vi "top地址搜索.vi"() -> ()   [LabVIEW 2020]
uses:
  e70b21cd-6488-4bde-bb2b-1088b515f470.vi
  <vilib>/Utility/file.llb/Read Delimited Spreadsheet (string).vi
  <vilib>/Comparison/Equal/Equal Functor/Equal Functor.lvclass
panel:
  in  "file path (dialog if empty) 2":path=path "D:/NI 资源包/2-币猎人-事件状态机930/source/规则大数.txt" caption="文件路径 （空时为对话框）"
  out "子数组 3":string[](array[string])
  out "子数组 2":string[](array[string])
  out "数值 2":i32
  out "添加的路径":path
  in  "停止":bool
  out "地址":string
  out "数组":string[][](array[string])
  out "数值":i32
  out "文件名":string[](array[string])
  out "路径输出":path
  in  "路径":path=path "D:/NI 资源包/2-币猎人-事件状态机930/source/网址私钥获取/btc搜寻器/top 账号数据"
  out "index of element":i32 caption="元素索引"
  out "子数组":string[](array[string])
  out "all rows":string[][](array[string]) caption="所有行"
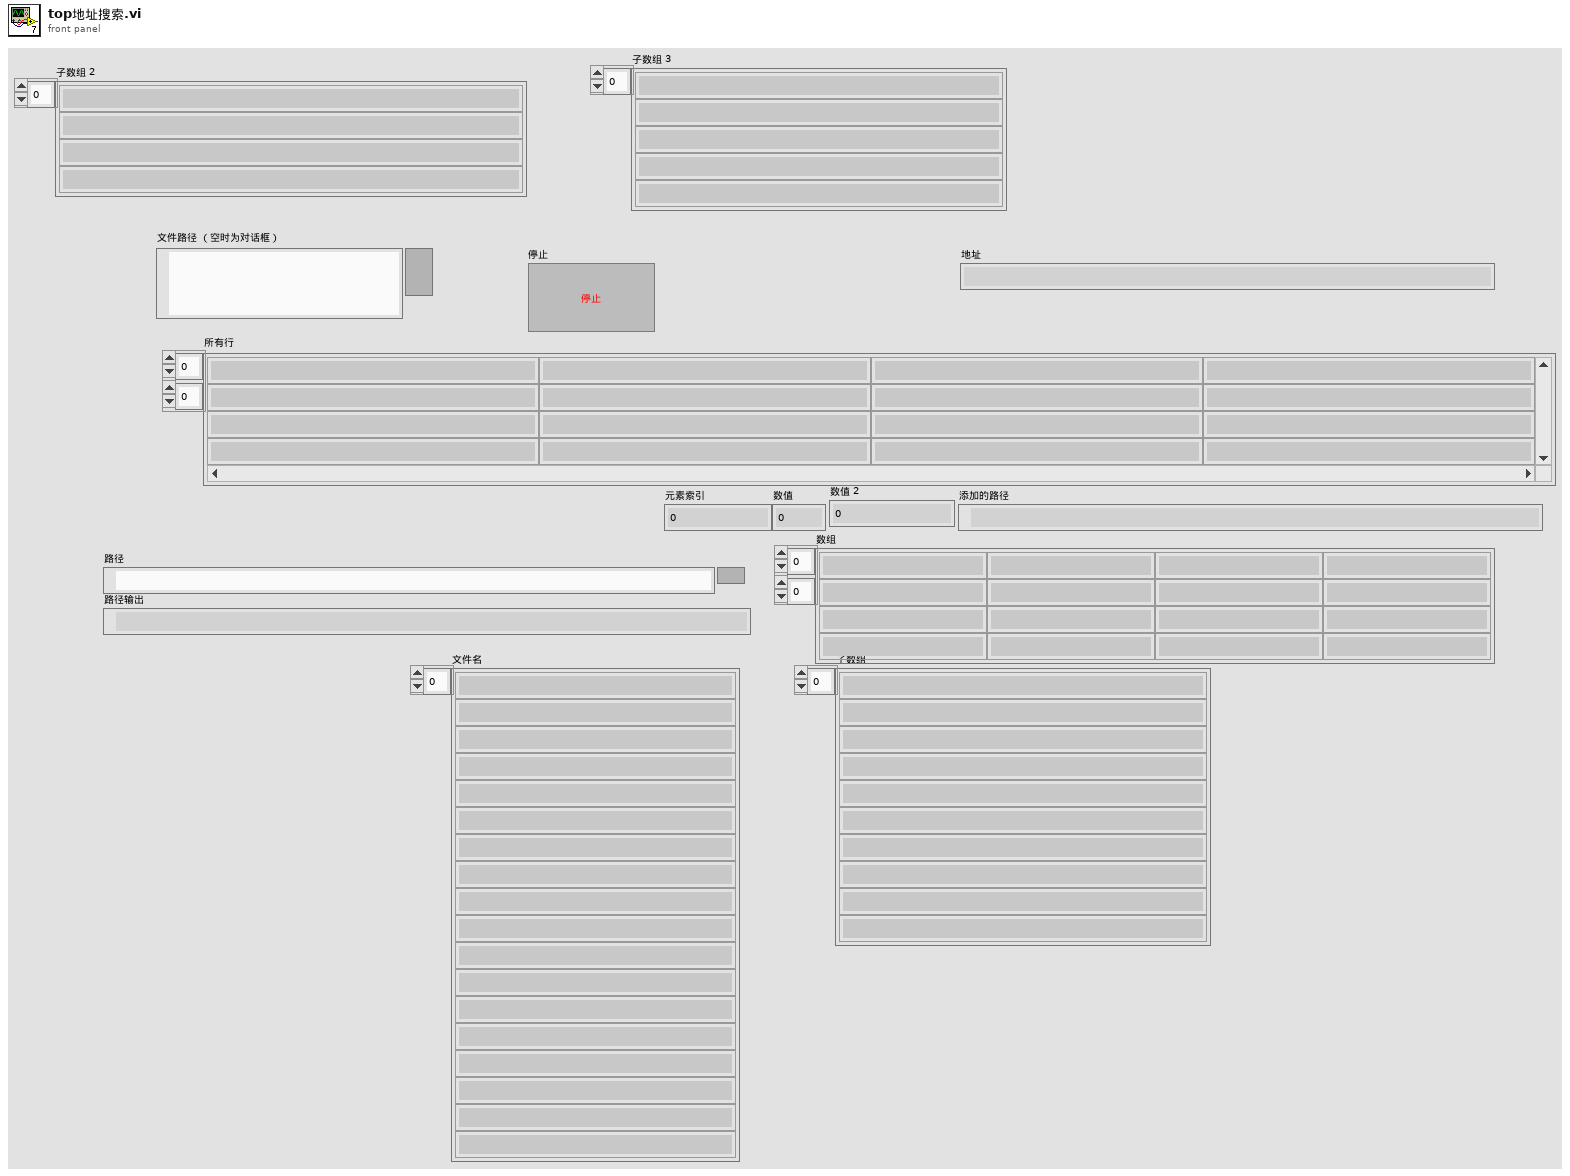
[diagram p1: front panel]
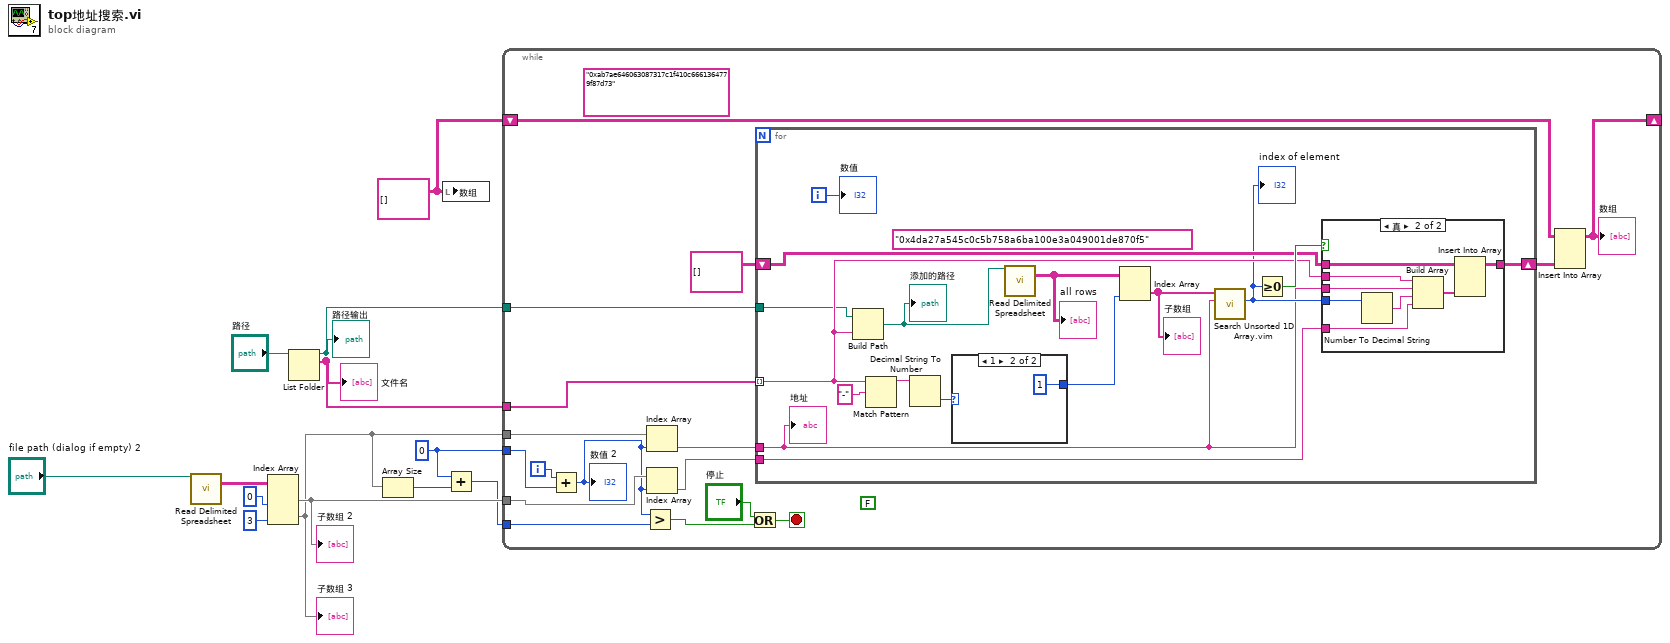
[diagram p0: block diagram]
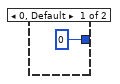
[diagram p3: hidden frame]
diagram:
  w6 = 0 ("y")
  w13 = string[][] []
  n1 = call-poly <vilib>:"Read Delimited Spreadsheet.vi"("file path (dialog if empty)"="file path (dialog if empty) 2") -> ("all rows"=w9:string[][])  [unwired: 9 in, 5 out]
  n2 = Index Array(array=w9, index (col) #1=0 ("禁用的索引 (列)"), index (col) #2=3 ("索引 (列)")) -> (element #1=w8:string[], element #2=w7:string[])  [unwired: 2 in]
  "子数组 2" <- w8
  "子数组 3" <- w7
  n3 = List Folder(path="路径") -> (path out=w1:path, filenames=w2:string[])  [unwired: 3 in, 2 out]
  "路径输出" <- w1
  "文件名" <- w2
  n4 = Array Size(array=w7) -> (size(s)=w5:i32)
  n5 = local write "数组"(w13) -> ()
  n6 = Add(x=w6, y=w5) -> (x+y=w4:i32)
  n7 = while {
    shift-right: [w27] -> _
    shift-left: w13 -> [w29]
    tunnel: w7 -> [w21]
    tunnel: w8 -> [w23]
    tunnel: w6 -> [w19]
    tunnel: w4 -> [w17]
    tunnel: w2 -> [w15]
    tunnel: w1 -> [w14]
    i -> [w24]
    stop <- w25 stop-if-true
    (unwired) FALSE ("y")
    (unwired) "0xab7ae646063087317c1f410c6661364779f87d73" ("地址")
    n8 = Add(x=w24, y=w19) -> (x+y=w18:i32)
    "数值 2" <- w18
    n9 = Greater?(x=w18, y=w17) -> (0:w16:bool)
    n10 = Index Array(array=w21, index=w18) -> (element=w20:string)
    n11 = Index Array(array=w23, index=w18) -> (element=w22:string)
    n12 = Or(x="停止", y=w16) -> (x .or. y?=w25:bool)
    n13 = for {
      tunnel: w15 -> [w36] mode=indexing
      shift-right: [w34] -> w28
      shift-left: string[][] [] -> [w37]
      tunnel: w22 -> [w32]
      tunnel: w20 -> [w33]
      tunnel: w14 -> [w31]
      i -> [w39]
      (unwired) "0x4da27a545c0c5b758a6ba100e3a049001de870f5" ("元素 2")
      n14 = Build Path(base path=w31, name or relative path=w36) -> (appended path=w40:path)
      "添加的路径" <- w40
      n15 = Match Pattern(string=w36, regular expression="-" ("正则表达式")) -> (before substring=w45:string)  [unwired: 1 in, 3 out]
      n16 = Decimal String To Number(string=w45) -> (number=w44:i32)  [unwired: 2 in, 1 out]
      n17 = case shown="1" w44 {
        tunnel: [0 ("禁用的索引 (列)") 1 ("禁用的索引 (列)")] -> w41
        frame 0, Default {
        }
        frame 1 {
        }
      }
      n18 = call-poly <vilib>:"Read Delimited Spreadsheet.vi"("file path (dialog if empty)"=w40) -> ("all rows"=w42:string[][])  [unwired: 9 in, 5 out]
      "all rows" <- w42
      n19 = Index Array(array=w42, index (col)=w41) -> (element=w43:string[])  [unwired: 1 in]
      "子数组" <- w43
      n20 = call "Search Unsorted 1D Array.vim"("element"=w33, "unsorted 1D array"=w43) -> ("index of element"=w35:i32)  [unwired: 9 in]
      "index of element" <- w35
      n21 = Greater Or Equal To 0?(x=w35) -> (x >= 0?=w38:bool)
      n22 = case shown="真" w38 {
        tunnel: w33 -> [_ w49]
        tunnel: w37 -> [w47 w53]
        tunnel: w36 -> [_ w50]
        tunnel: w35 -> [_ w55]
        tunnel: [w47 w51] -> w34
        tunnel: w32 -> [_ w48]
        frame False {
        }
        frame True {
          n23 = Number To Decimal String(number=w55) -> (decimal integer string=w54:string)  [unwired: 1 in]
          n24 = Build Array(w50, w49, w54, w48) -> (w52:string[])
          n25 = Insert Into Array(array=w53, new element=w52) -> (w51:string[][])  [unwired: 2 in]
        }
      }
      "数值" <- w39
      "地址" <- w33
    }
    n26 = Insert Into Array(array=w29, new element=w28) -> (w27:string[][])  [unwired: 2 in]
    "数组" <- w27
  }
